vi "Connect_PSU_GCFS.vi"(4 "error in (no error)":errorcluster, 7 "?":T1 {"Data Out Cluster"."Particle Measurements" format="%.2f"}) -> (0 "error out":errorcluster, 1 "State out":string, 2 "Connected?":bool, 3 "output cluster":T1={"Core"={"Current VI Reference"=refnum, "Close Panel on Exit?"=FALSE}, "Your Boolean data"=FALSE, "Your string data"="", "Camera Cluster"={"Session"="", "Image"=refnum, "Position Image"=refnum, "PixelVal Image"=refnum, "Position Image Binary"=refnum, "Lable Image"=refnum, "Merged Image"=refnum}, "Data In Cluster"={"Images"={"Position Image path"=path "", "Sample folder path"=path "", "Label Image path"=path ""}, "Sample Name"="", "Sample Rate"=20, "Gradient Buffer"=0, "Data Acquisition.Setup.TempGrad"=0.0, "Control.PID gains"={"proportional gain (Kc)"=0.0, "integral time (Ti, min)"=0.0, "derivative time (Td, min)"=0.0}}, "Active"=FALSE, "Ready"=FALSE, "Exit"=FALSE, "Arduino"={"Connection"=FALSE, "Port"="", "State"=""}, "Program_Start"="", "Data Out Cluster"={"Particle Measurements"=[], "Number of droplets"=0, "PosImg_Timestamp"="", "OverlayProp"=[], "Group"="", "Que"=refnum}, "PSU"={"Connection"=FALSE, "Port"="", "State"=""}, "Load Rerun"=FALSE, "Rerun"=FALSE} {"Data Out Cluster"."Particle Measurements" format="%.2f"})   [LabVIEW 2024]
uses:
  Micro/DataCluster_GCFS.ctl
  <vilib>/userDefined/High Color/IMAQdx.ctl
  <vilib>/vision/Image Controls.llb/IMAQ Image.ctl
  <vilib>/vision/Image Controls.llb/Overlay Property.ctl
  3fecfa67-3b21-477e-abb9-e6c266c22bf3.vi
  c3f8f1ca-e765-4d6e-aaca-1dfa09713a13.vi
  f28ec6ae-94ae-46b8-8c3f-28958ce1d9fa.vi
  a9b37c8b-7b1a-4864-ae66-bc56c044b39d.vi
  <vilib>/regexp/Match Regular Expression.xnode
panel:
  out "Device describtion":string[](array[string])
  out "find list":string[](array[string])
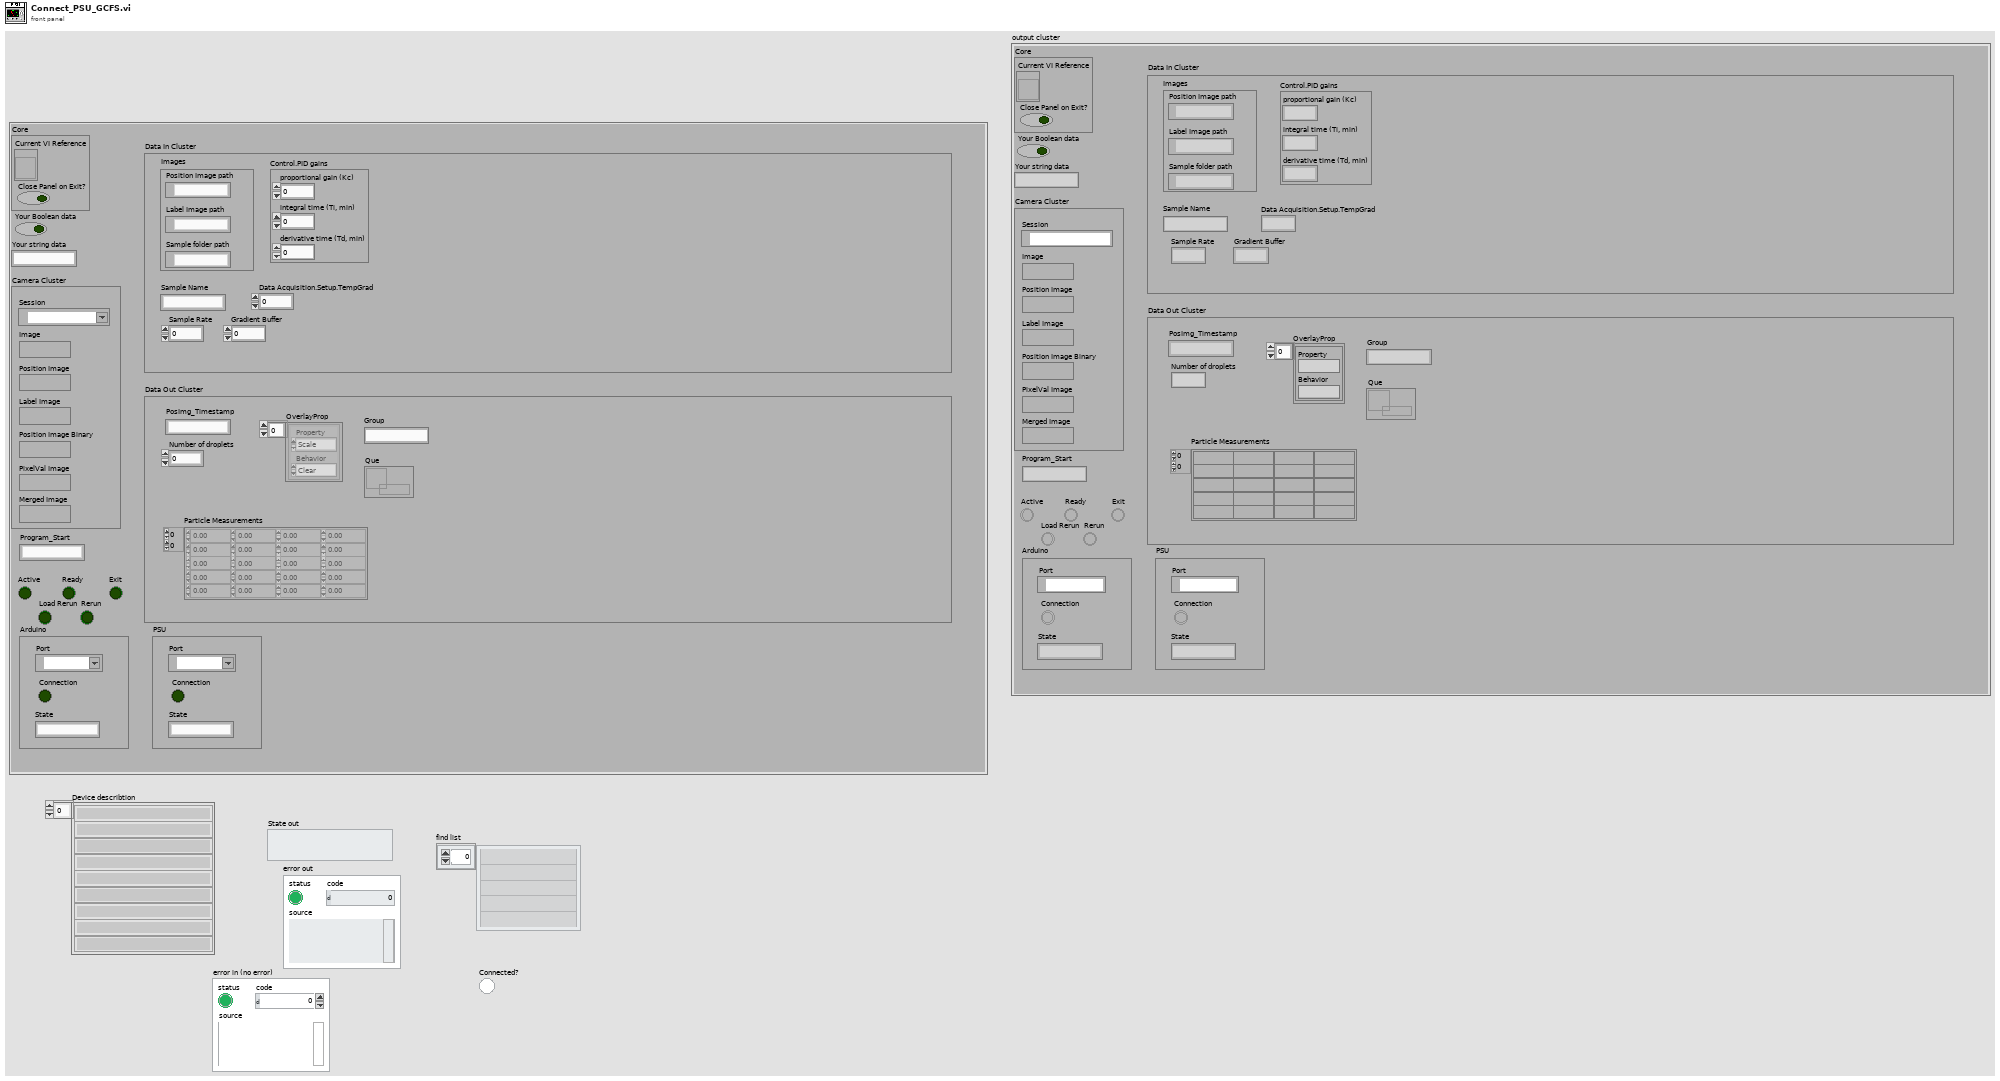
[diagram p1: front panel]
types:
  T1 = typedef "DataCluster_GCFS.ctl" = cluster{"Core":cluster{"Current VI Reference":refnum<vi>, "Close Panel on Exit?":bool}, "Your Boolean data":bool, "Your string data":string, "Camera Cluster":cluster{"Session":T2, "Image":T3, "Position Image":T3, "PixelVal Image":T3, "Position Image Binary":T3, "Lable Image":T3, "Merged Image":T3}, "Data In Cluster":cluster{"Images":cluster{"Position Image path":path, "Sample folder path":path, "Label Image path":path}, "Sample Name":string, "Sample Rate":i32, "Gradient Buffer":i32, "Data Acquisition.Setup.TempGrad":dbl, "Control.PID gains":cluster{"proportional gain (Kc)":dbl, "integral time (Ti, min)":dbl, "derivative time (Td, min)":dbl}}, "Active":bool, "Ready":bool, "Exit":bool, "Arduino":cluster{"Connection":bool, "Port":refnum<visa-resource-name>, "State":string}, "Program_Start":string, "Data Out Cluster":cluster{"Particle Measurements":dbl[][], "Number of droplets":i32, "PosImg_Timestamp":string, "OverlayProp":T4[], "Group":string, "Que":refnum<queue>}, "PSU":cluster{"Connection":bool, "Port":refnum<visa-resource-name>, "State":string}, "Load Rerun":bool, "Rerun":bool}
  T2 = typedef "IMAQdx.ctl" = refnum<k21>
  T3 = typedef "IMAQ Image.ctl" = refnum<image>
  T4 = typedef "Overlay Property.ctl" = cluster{"Property":enum32{"Scale", "Shift", "Rotate", "Symmetry"}, "Behavior":enum32{"Clear", "Keep", "Transform"}}
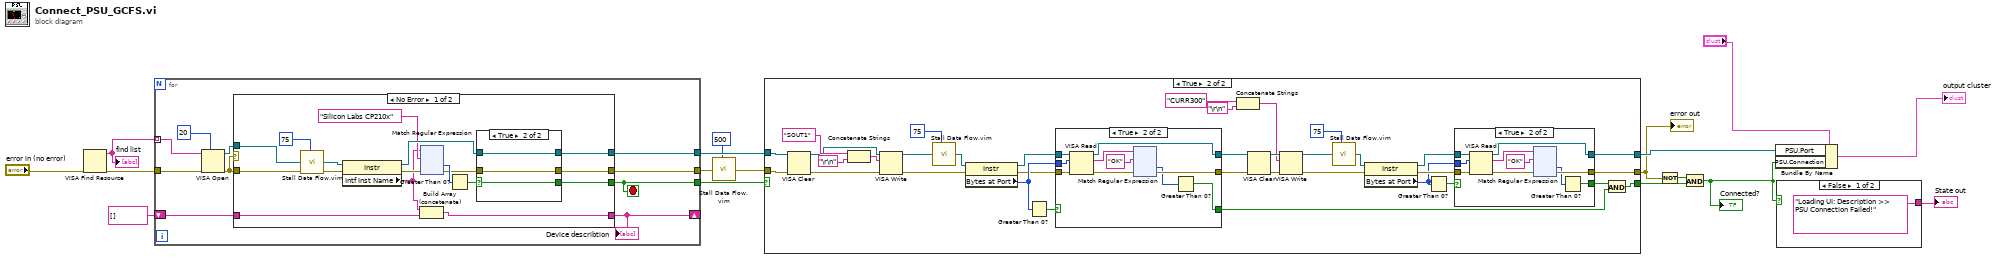
[diagram p0: block diagram]
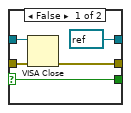
[diagram p3: hidden frame]
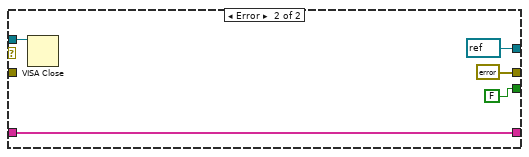
[diagram p4: hidden frame]
diagram:
  n1 = VISA Find Resource(8:"error in (no error)") -> (0:w16:errorcluster, 3:w17:string[])  [unwired: 2 in, 1 out]
  "find list" <- w17
  n2 = for {
    tunnel: w17 -> [w27] mode=indexing
    tunnel: w16 -> [w26]
    tunnel: [w23] -> w3
    tunnel: [w22] -> w14
    tunnel: [w24] -> w13
    shift-right: [w19] -> _
    shift-left: string[] [] -> [w18]
    stop <- w22 stop-if-true
    n3 = VISA Open(timeout (0)=u32 20 ("VISA Open timeout (0)"), error in (no error)=w26, VISA resource name=w27) -> (VISA resource name=w21:refnum<visa-resource-name>, error out=w25:errorcluster)  [unwired: 2 in]
    n4 = case shown="No Error" w25 {
      tunnel: w21 -> [w33 w171]
      tunnel: w25 -> [w43 _]
      tunnel: [w40 refnum<visa-resource-name> refnum ("Port")] -> w24
      tunnel: [w39 FALSE] -> w22
      tunnel: [w38 errorcluster {"status"=FALSE, "code"=0, "source"=""} ("error out")] -> w23
      tunnel: [w29 w169] -> w19
      tunnel: w18 -> [w28 w169]
      frame No Error {
        n5 = call "Stall Data Flow.vim"("value in"=w33, "milliseconds to wait"=u32 75) -> ("value out"=w32:refnum<visa-resource-name>)  [unwired: 1 out]
        n6 = property class="Instr"(reference=w32, error in=w43) -> (reference out=w41:refnum<visa-resource-name>, error out=w35:errorcluster, "Intf Inst Name"=w30:string)
        n7 = Build Array (concatenate)(w30, w28) -> (w29:string[])
        n8 = xnode "Match Regular Expression"("input string"=w30, "regular expression"="Silicon Labs CP210x", "error in"=w35) -> ("offset past match"=w36:i32, "error out"=w34:errorcluster)  [unwired: 3 in, 3 out]
        n9 = Greater Than 0?(x=w36) -> (x > 0?=w42:bool)
        n10 = case shown="True" w42 {
          selector: w42 -> [w165 w167]
          tunnel: w41 -> [w164 w168]
          tunnel: [refnum<visa-resource-name> refnum ("Port") w168] -> w40
          tunnel: [w165 w167] -> w39
          tunnel: w34 -> [w163 w166]
          tunnel: [w162 w166] -> w38
          frame False {
            n11 = VISA Close(VISA resource name=w164, error in (no error)=w163) -> (error out=w162:errorcluster)
          }
          frame True {
          }
        }
      }
      frame Error {
        n12 = VISA Close(VISA resource name=w171) -> ()  [unwired: 1 in, 1 out]
      }
    }
    "Device describtion" <- w19
  }
  n13 = call "Stall Data Flow.vim"("value in"=w3, "milliseconds to wait"=u32 500) -> ("value out"=w2:errorcluster)  [unwired: 1 out]
  n14 = case shown="True" w14 {
    selector: w14 -> [w175 _]
    tunnel: w13 -> [w174 w208]
    tunnel: w2 -> [w176 w207]
    tunnel: [w174 w179] -> w12
    tunnel: [w176 w180] -> w9
    tunnel: [w175 w178] -> w11
    frame False {
    }
    frame True {
      n15 = VISA Clear(VISA resource name=w208, error in (no error)=w207) -> (VISA resource name out=w206:refnum<visa-resource-name>, error out=w205:errorcluster)
      n16 = Concatenate Strings("SOUT1" ("string"), "\r\n") -> (w209:string)
      n17 = VISA Write(VISA resource name=w206, write buffer=w209, error in (no error)=w205) -> (VISA resource name out=w198:refnum<visa-resource-name>, error out=w197:errorcluster)  [unwired: 1 out]
      n18 = call "Stall Data Flow.vim"("value in"=w198, "milliseconds to wait"=u32 75) -> ("value out"=w204:refnum<visa-resource-name>)  [unwired: 1 out]
      n19 = property class="Instr"(reference=w204, error in=w197) -> (reference out=w201:refnum<visa-resource-name>, error out=w200:errorcluster, "Bytes at Port"=w202:u32)
      n20 = Greater Than 0?(x=w202) -> (x > 0?=w203:bool)
      n21 = case shown="True" w203 {
        selector: w203 -> [w342 _]
        tunnel: w202 -> [_ w354]
        tunnel: w200 -> [w343 w353]
        tunnel: [w344 w352] -> w182
        tunnel: [w343 w347] -> w181
        tunnel: w201 -> [w344 w351]
        tunnel: [w342 w345] -> w196
        frame False {
        }
        frame True {
          n22 = VISA Read(VISA resource name=w351, byte count=w354, error in (no error)=w353) -> (VISA resource name out=w352:refnum<visa-resource-name>, read buffer=w350:string, error out=w349:errorcluster)  [unwired: 1 out]
          n23 = xnode "Match Regular Expression"("input string"=w350, "regular expression"="OK", "error in"=w349) -> ("offset past match"=w346:i32, "error out"=w347:errorcluster)  [unwired: 3 in, 3 out]
          n24 = Greater Than 0?(x=w346) -> (x > 0?=w345:bool)
        }
      }
      n25 = Concatenate Strings("CURR300" ("string"), "\r\n") -> (w186:string)
      n26 = VISA Clear(VISA resource name=w182, error in (no error)=w181) -> (VISA resource name out=w187:refnum<visa-resource-name>, error out=w188:errorcluster)
      n27 = VISA Write(VISA resource name=w187, write buffer=w186, error in (no error)=w188) -> (VISA resource name out=w194:refnum<visa-resource-name>, error out=w195:errorcluster)  [unwired: 1 out]
      n28 = call "Stall Data Flow.vim"("value in"=w194, "milliseconds to wait"=u32 75) -> ("value out"=w189:refnum<visa-resource-name>)  [unwired: 1 out]
      n29 = property class="Instr"(reference=w189, error in=w195) -> (reference out=w192:refnum<visa-resource-name>, error out=w193:errorcluster, "Bytes at Port"=w191:u32)
      n30 = Greater Than 0?(x=w191) -> (x > 0?=w190:bool)
      n31 = case shown="True" w190 {
        selector: w190 -> [w212 _]
        tunnel: w191 -> [_ w224]
        tunnel: w193 -> [w213 w223]
        tunnel: [w214 w222] -> w179
        tunnel: [w213 w217] -> w180
        tunnel: w192 -> [w214 w221]
        tunnel: [w212 w215] -> w177
        frame False {
        }
        frame True {
          n32 = VISA Read(VISA resource name=w221, byte count=w224, error in (no error)=w223) -> (VISA resource name out=w222:refnum<visa-resource-name>, read buffer=w220:string, error out=w219:errorcluster)  [unwired: 1 out]
          n33 = xnode "Match Regular Expression"("input string"=w220, "regular expression"="OK", "error in"=w219) -> ("offset past match"=w216:i32, "error out"=w217:errorcluster)  [unwired: 3 in, 3 out]
          n34 = Greater Than 0?(x=w216) -> (x > 0?=w215:bool)
        }
      }
      n35 = And(x=w177, y=w196) -> (x .and. y?=w178:bool)
    }
  }
  "error out" <- w9
  n36 = Not(x=w9) -> (.not. x?=w7:bool)
  n37 = And(x=w7, y=w11) -> (x .and. y?=w8:bool)
  "Connected?" <- w8
  n38 = Bundle By Name(cluster="?", "PSU.Port"=w12, "PSU.Connection"=w8) -> (→"output cluster":T1)
  n39 = case shown="False" w8 {
    tunnel: ["Loading UI: Description >> PSU Connection Failed!" _] -> w10
    frame False {
    }
    frame True {
    }
  }
  "State out" <- w10
